vi "oldBallToOOBall.vi"(8 "error in (no error)":errorcluster, 9 "SSL_BallModelStraightTwoPhase":T1, 10 "balls":T2[](array[typedef]), 11 "Ball in":refnum<class "Ball.lvclass">) -> (0 "error out":errorcluster, 3 "Ball out":refnum<class "Ball.lvclass">)   [LabVIEW 2023, in "Ball.lvclass"]
uses:
  Ball.lvclass
  C:/Users/lucio/Desktop/roboime/SSL_AI/Object_class/Object.lvclass
  Vision_class/Old vision/SSL Detection Frame Simple Estimator Cameras VelCmd Folder/Core/AI Ball.ctl
  Vision_class/Old vision/Controls/SSL_BallModelStraightTwoPhase.ctl
  Ball.lvclass/Ball.ctl
  Object_class/Object.lvclass/Object.ctl
  Write z.vi
  Object_class/Write x.vi
  Object_class/Write y.vi
  Write v_x.vi
  Write v_y.vi
  Object_class/Write pos_est_x.vi
  Object_class/Write pos_est_y.vi
  Write Valid.vi
  Write Existent.vi
  Write acc_slide.vi
  Write acc_roll.vi
  Write k_switch.vi
  Vision_class/Vision.lvclass
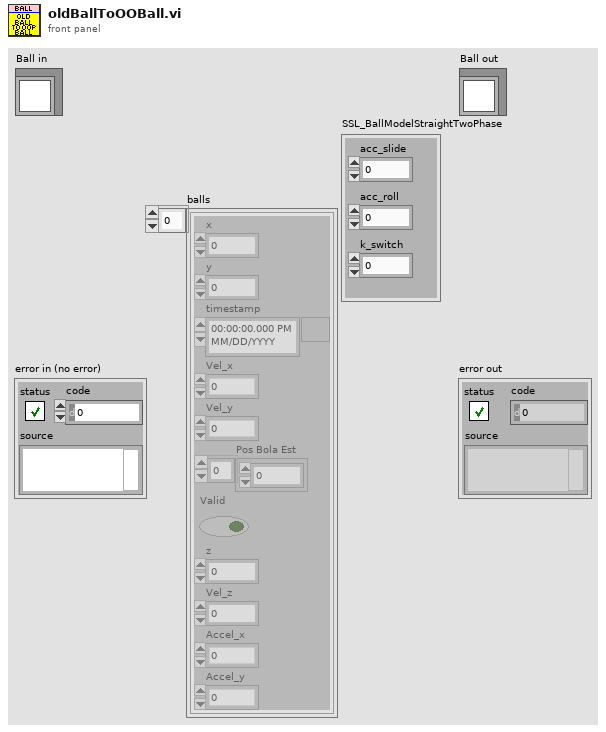
[diagram p1: front panel]
types:
  T1 = typedef "Vision.lvclass/SSL_BallModelStraightTwoPhase.ctl" = cluster{"acc_slide":dbl, "acc_roll":dbl, "k_switch":dbl}
  T2 = typedef "AI Ball.ctl" = cluster{"x":dbl, "y":dbl, "timestamp":timestamp, "Vel_x":dbl, "Vel_y":dbl, "Pos Bola Est":dbl[], "Valid":bool, "z":dbl, "Vel_z":dbl, "Accel_x":dbl, "Accel_y":dbl}
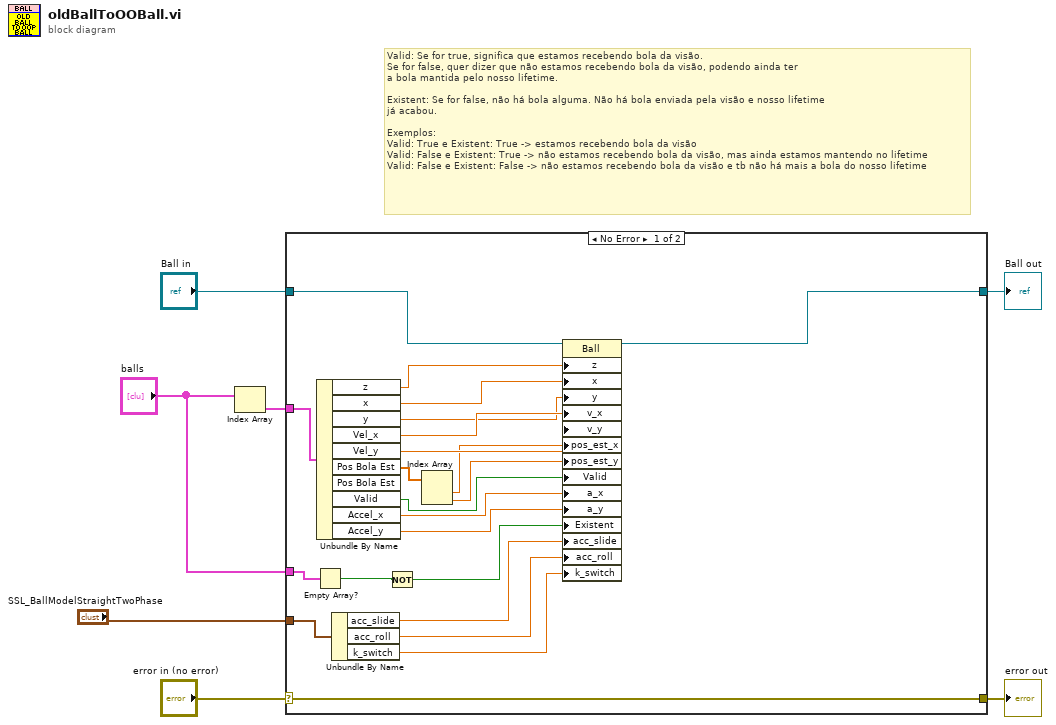
[diagram p0: block diagram]
diagram:
  # "Valid: Se for true, significa que estamos recebendo bola da visão.\nSe for false, quer dizer que não estamos recebendo bola da visão, podendo ainda ter\na bola mantida pelo nosso lifetime.\n\nExistent: Se for false, não há bola alguma. Não há bola enviada pela visão e nosso lifetime\njá acabou.\n\nExemplos:\nValid: True e Existent: True -> estamos recebendo bola da visão\nValid: False e Existent: True -> não estamos recebendo bola da visão, mas ainda estamos mantendo no lifetime\nValid: False e Existent: False -> não estamos recebendo bola da visão e tb não há mais a bola do nosso lifetime"
  n1 = Index Array(array="balls") -> (element=w3:T2)  [unwired: 1 in]
  n2 = case shown="No Error" "error in (no error)" {
    selector: "error in (no error)" -> [w29 w31]
    tunnel: [w29 w31] -> w6
    tunnel: [w10 w30] -> w4
    tunnel: "Ball in" -> [w28 w30]
    tunnel: w3 -> [w27 _]
    tunnel: "balls" -> [w20 _]
    tunnel: "SSL_BallModelStraightTwoPhase" -> [w14 _]
    frame No Error {
      n3 = Empty Array?(array=w20) -> (empty?=w18:bool)
      n4 = Unbundle By Name(w27) -> ("z"=w21:dbl, "x"=w9:dbl, "y"=w8:dbl, "Vel_x"=w26:dbl, "Vel_y"=w25:dbl, "Pos Bola Est"=w24:dbl[], "Valid"=w19:bool, "Accel_x"=w16:dbl, "Accel_y"=w15:dbl)  [unwired: 1 out]
      n5 = Unbundle By Name(w14) -> ("acc_slide"=w13:dbl, "acc_roll"=w11:dbl, "k_switch"=w12:dbl)
      n6 = Not(x=w18) -> (.not. x?=w17:bool)
      n7 = Index Array(array=w24) -> (element #1=w23:dbl, element #2=w22:dbl)  [unwired: 2 in]
      n8 = property class="Ball"(reference=w28, "z"=w21, "x"=w9, "y"=w8, "v_x"=w26, "v_y"=w25, "pos_est_x"=w23, "pos_est_y"=w22, "Valid"=w19, "a_x"=w16, "a_y"=w15, "Existent"=w17, "acc_slide"=w13, "acc_roll"=w11, "k_switch"=w12) -> (reference out=w10:refnum<class "Ball.lvclass">)  [unwired: 1 in, 1 out]
    }
    frame Error {
    }
  }
  "error out" <- w6
  "Ball out" <- w4
